vi "Instr_SetPrivateData.vi"(8 "error in (no error)":errorcluster, 11 "MultimeterControl in":refnum<class "MultimeterControl.lvclass">) -> (0 "error out":errorcluster, 3 "MultimeterControl out":refnum<class "MultimeterControl.lvclass">)   [LabVIEW 2013, in "MultimeterControl.lvclass"]
uses:
  MultimeterControl.lvclass
  InstrControl.lvclass
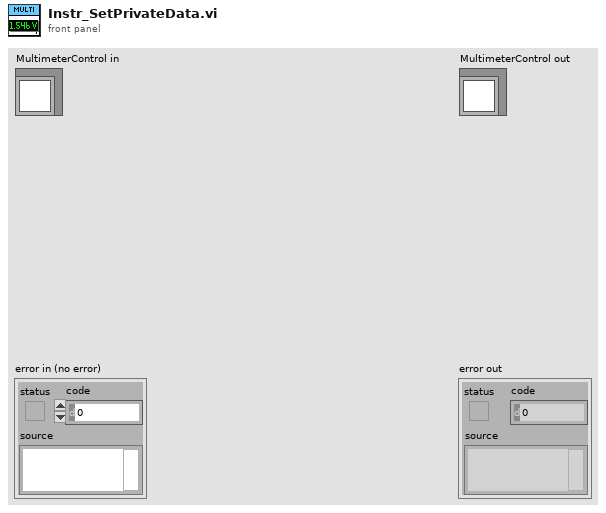
[diagram p1: front panel]
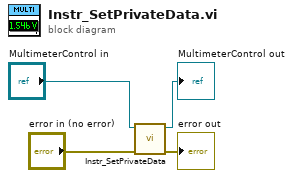
[diagram p0: block diagram]
diagram:
  n1 = call-parent "Instr_SetPrivateData.vi"("error in (no error)"="error in (no error)", "InstrControl in"="MultimeterControl in") -> ("error out"=→"error out":errorcluster, "InstrControl out"=→"MultimeterControl out":refnum<class "MultimeterControl.lvclass">)  [unwired: 8 in]
